vi "Global_SEN_Data Out.vi"() -> ()   [LabVIEW 2023, in "PigeonIMU w Tilt_SEN.lvlib"]
uses:
  PigeonIMU w Tilt_SEN.lvlib
  Shared Code/TypeDefs/Cluster_Unity Yaw-Pitch-Roll.ctl
  Shared Code/TypeDefs/Dial_Compase heading unit circle CCW positive.ctl
  Type Defs/Cluster_Yaw Pitch Roll in Deg.ctl
  Type Defs/Cluster_Pigeon Tilt Data.ctl
  Shared Code/TypeDefs/ENUM_Tilt State.ctl
panel:
  out "Sen_Pigeon_Tilt Data":T1
  out "Sen_Pigeon_YawPitchRoll(deg)":T3
  out "Sen_Pigeon_Swinging":bool
  out "Sen_Pigeon_Running":bool
  out "Sen_Pigeon_YawPitchRoll":T4 {"Roll" scale format="%.3f"; "Pitch" scale format="%.3f"; "Yaw" scale format="%.3f"}
  # "The Names of the Data items in the Global Variable MUST describe who the Single Writer is\nFor Sensor Globals the the naming convention is\n   \nSEN_Lib Name_Data Name\n\nExamples:\nSEN_Gyro_Angle\nSEN_Sonar_Distance"
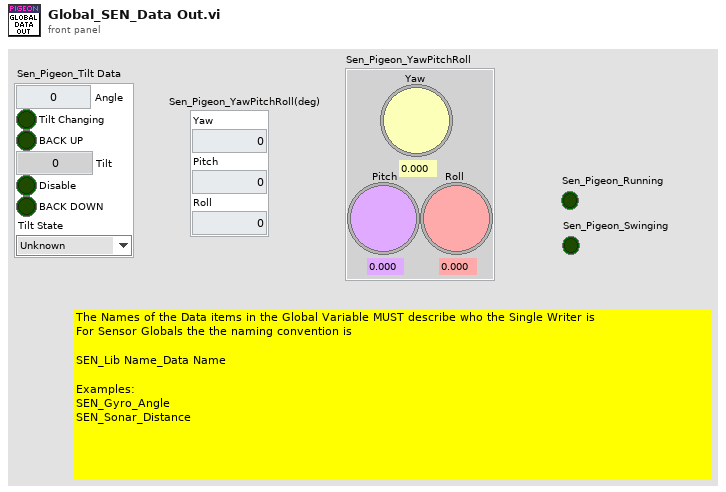
[diagram p1: front panel]
types:
  T1 = typedef "Cluster_Pigeon Tilt Data.ctl" = cluster{"Angle":dbl, "Tilt Changing":bool, "BACK UP":bool, "Tilt":dbl, "Disable":bool, "BACK DOWN":bool, "Tilt State":T2}
  T2 = typedef "ENUM_Tilt State.ctl" = enum16{"Unknown", "Level", "Angle UP from Level", "Level from Angle Up", "Angle Down from Level", "Level from Angle Down"}
  T3 = typedef "Cluster_Yaw Pitch Roll in Deg.ctl" = cluster{"Yaw":dbl, "Pitch":dbl, "Roll":dbl}
  T4 = typedef "Cluster_Unity Yaw-Pitch-Roll.ctl" = cluster{"Yaw":T5, "Pitch":T5, "Roll":T5}
  T5 = typedef "Dial_Compase heading unit circle CCW positive.ctl" = dbl
diagram:
